vi "Sequence Check Operation Enable.vi"(10 "System State":map{string, dbl}(c390), 11 "Sequencer Data Context IN":T1={"Sequencer State"=enum."Clear Drive Fault", "Event Timeout"=-1, "Current Index"=0, "Sequence Timeout"=0, "Turbine RPM Array"=[], "Pump RPM Array"=[], "Duration (Seconds) Array"=[], "Folder Path"=path ""}) -> (3 "Sequencer Data Context OUT":T1={"Sequencer State"=enum."Clear Drive Fault", "Event Timeout"=-1, "Current Index"=0, "Sequence Timeout"=0, "Turbine RPM Array"=[], "Pump RPM Array"=[], "Duration (Seconds) Array"=[], "Folder Path"=path ""})   [LabVIEW 2024, in "Auto Modo.lvlib"]
uses:
  Auto Modo.lvlib
  Sequencer Data Context.ctl
  Sequencer State.ctl
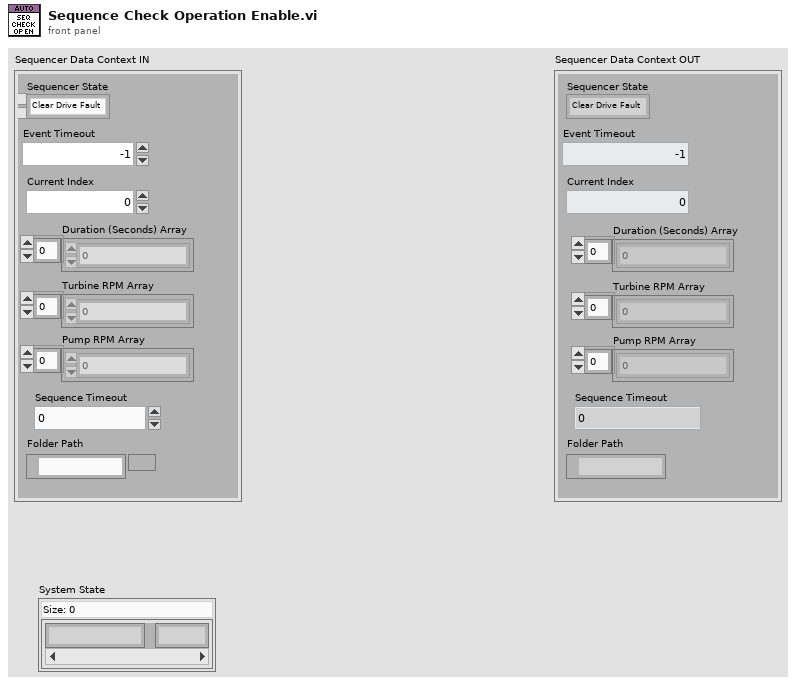
[diagram p1: front panel]
types:
  T1 = typedef "Auto Modo.lvlib/Sequencer Data Context.ctl" = cluster{"Sequencer State":T2, "Event Timeout":i32, "Current Index":i32, "Sequence Timeout":i32, "Turbine RPM Array":dbl[], "Pump RPM Array":dbl[], "Duration (Seconds) Array":dbl[], "Folder Path":path}
  T2 = typedef "Auto Modo.lvlib/Sequencer State.ctl" = enum16{"Idle", "Initial Check Enable Operation", "Clear Drive Fault", "Check Drive Fault", "Set Ready to Switch ON", "Check Ready to Switch ON", "Enable Operation", "Check Enable Operation", "Set Drive RPM", "Check Drive RPM", "Next Drive RPM", "Final"}
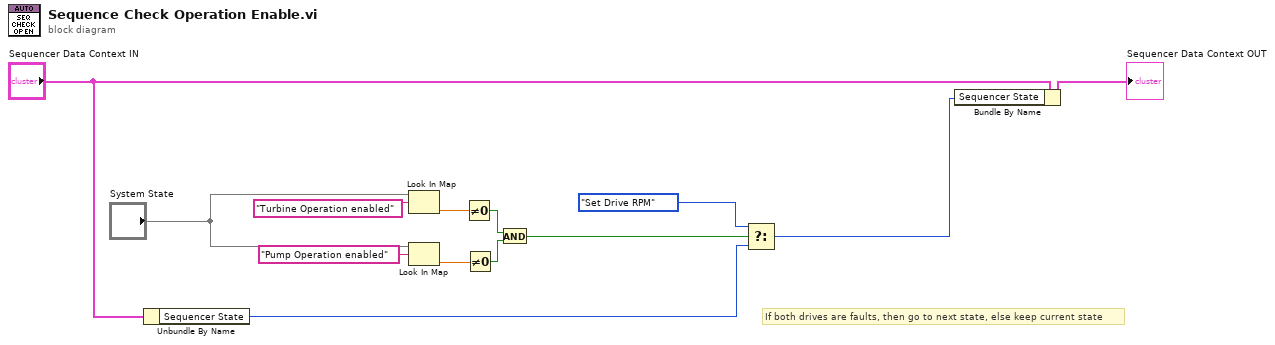
[diagram p0: block diagram]
diagram:
  # "If both drives are faults, then go to next state, else keep current state"
  n1 = Unbundle By Name("Sequencer Data Context IN") -> ("Sequencer State"=w1:T2)
  n2 = Look In Map(map="System State", key="Turbine Operation enabled") -> (value=w11:dbl)  [unwired: 1 in, 1 out]
  n3 = Look In Map(map="System State", key="Pump Operation enabled") -> (value=w10:dbl)  [unwired: 1 in, 1 out]
  n4 = Not Equal To 0?(x=w11) -> (x != 0?=w9:bool)
  n5 = Not Equal To 0?(x=w10) -> (x != 0?=w8:bool)
  n6 = And(x=w9, y=w8) -> (x .and. y?=w6:bool)
  n7 = Select(t=Sequencer_State."Set Drive RPM" ("Sequencer State"), s=w6, f=w1) -> (s? t:f=w3:T2)
  n8 = Bundle By Name(cluster="Sequencer Data Context IN", "Sequencer State"=w3) -> (→"Sequencer Data Context OUT":T1)
